vi "Cal RHS (VIRef).vi"(8 "error in (no error)":errorcluster, 10 "RHS in":variant, 11 "Domain_Steady_2D_Polygon in":refnum<class "NI_Domain_Steady_2D_Polygon.lvclass">) -> (0 "error out":errorcluster, 2 "RHS out":variant, 3 "Domain_Steady_2D_Polygon out":refnum<class "NI_Domain_Steady_2D_Polygon.lvclass">)   [LabVIEW 2017, in "NI_PDE.lvlib" / "NI_Domain_Steady_2D_Polygon.lvclass"]
uses:
  <vilib>/gmath/pde.llb/DomainClass/Domain_Steady_2D_Polygon/NI_Domain_Steady_2D_Polygon.lvclass
  <vilib>/gmath/pde.llb/RHSClass/RHS_2D_VIRef/RHS Data.ctl
  <vilib>/gmath/pde.llb/DomainClass/Domain_Steady_2D_Polygon/NI_Domain_Steady_2D_Polygon.lvclass/NI_Domain_Steady_2D_Polygon.ctl
  <vilib>/gmath/pde.llb/RHSClass/RHS_2D_VIRef/NI_RHS_2D_VIRef.lvclass
  <vilib>/gmath/NI_PDE.lvlib
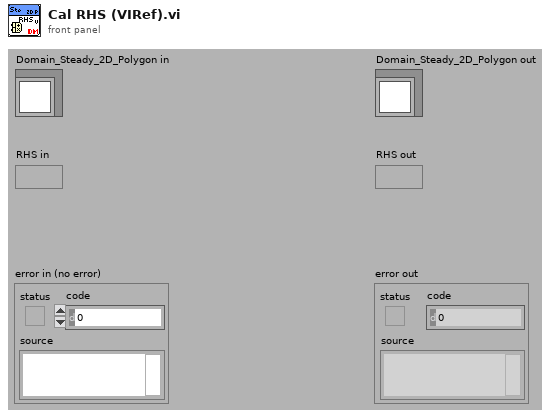
[diagram p1: front panel]
types:
  T1 = typedef "NI_PDE.lvlib/NI_RHS_2D_VIRef.lvclass/RHS Data.ctl" = cluster{"F":refnum<vi>, "data":variant}
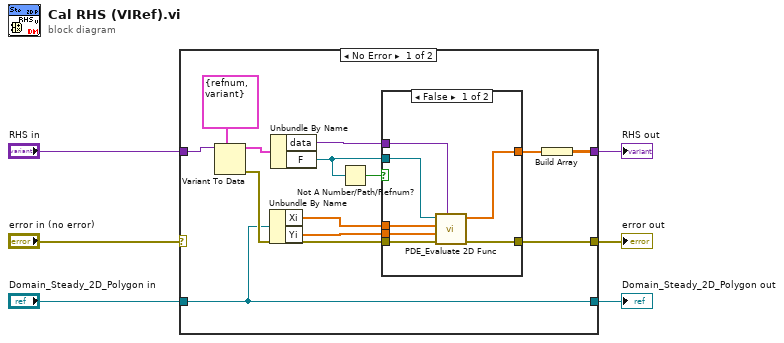
[diagram p0: block diagram]
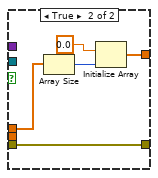
[diagram p2: hidden frame]
diagram:
  n1 = case shown="No Error" "error in (no error)" {
    selector: "error in (no error)" -> [_ w34]
    tunnel: "Domain_Steady_2D_Polygon in" -> [w7 w33]
    tunnel: [w7 w33] -> w6
    tunnel: [w11 w34] -> w5
    tunnel: [w12 w32] -> w2
    tunnel: "RHS in" -> [w19 w32]
    frame No Error {
      n2 = Variant To Data(type=T1 {"F"=refnum, "data"=variant} ("RHS data"), Variant=w19) -> (data=w13:T1, error out=w8:errorcluster)  [unwired: 1 in]
      n3 = Unbundle By Name(w7) -> ("Xi"=w10:dbl[], "Yi"=w9:dbl[])
      n4 = Unbundle By Name(w13) -> ("data"=w16:variant, "F"=w15:refnum<vi>)
      n5 = Not A Number/Path/Refnum?(number/path/refnum=w15) -> (NaN/Path/Refnum?=w14:bool)
      n6 = case shown="False" w14 {
        tunnel: w15 -> [w26 _]
        tunnel: w16 -> [w25 _]
        tunnel: w8 -> [w23 w30]
        tunnel: [w22 w30] -> w11
        tunnel: [w24 w28] -> w17
        tunnel: w10 -> [w21 w27]
        tunnel: w9 -> [w20 _]
        frame False {
          n7 = call <vilib>:"PDE_Evaluate 2D Func.vi"("data"=w25, "error in (no error)"=w23, "Y"=w20, "X"=w21, "VIRef"=w26) -> ("error out"=w22:errorcluster, "F(x, y)"=w24:dbl[])  [unwired: 5 out]
        }
        frame True {
          n8 = Array Size(array=w27) -> (size(s)=w29:i32)
          n9 = Initialize Array(0.0 ("element"), w29) -> (w28:dbl[])
        }
      }
      n10 = Build Array(w17) -> (w12:dbl[][])
    }
    frame Error {
    }
  }
  "Domain_Steady_2D_Polygon out" <- w6
  "error out" <- w5
  "RHS out" <- w2
